vi "Polynomial GCD Pair.vi"   [LabVIEW 2020, in "NI_AALPro.lvlib"]
uses:
  <vilib>/Analysis/NI_AALPro.lvlib
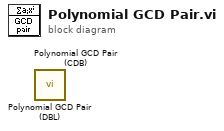
[diagram p0: block diagram]
diagram:
  n1 = call <vilib>:"Polynomial GCD Pair (DBL).vi"() -> ()  [unwired: 8 in, 4 out]
  n2 = call <vilib>:"Polynomial GCD Pair (CDB).vi"() -> ()  [unwired: 8 in, 4 out]
